vi "Areotech set positon.vi"(8 "error in (no error)":errorcluster, 10 "Parsed CMD":T1, 11 "AerotechStage in":refnum<class "AerotechStage.lvclass">) -> (0 "error out":errorcluster, 2 "new commands":string, 3 "AerotechStage out":refnum<class "AerotechStage.lvclass">)   [LabVIEW 2013, in "AerotechStage.lvclass"]
uses:
  AerotechStage.lvclass
  shared/parsed device cmd.ctl
  AerotechStage.lvclass/AerotechStage.ctl
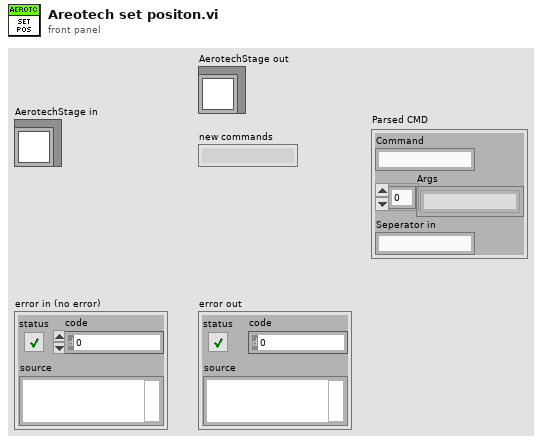
[diagram p1: front panel]
types:
  T1 = typedef "parsed device cmd.ctl" = cluster{"Command":string, "Args":string[], "Seperator in":string}
  T2 = typedef "OnOffTypeDef.ctl" = enum16{"off", "on"}
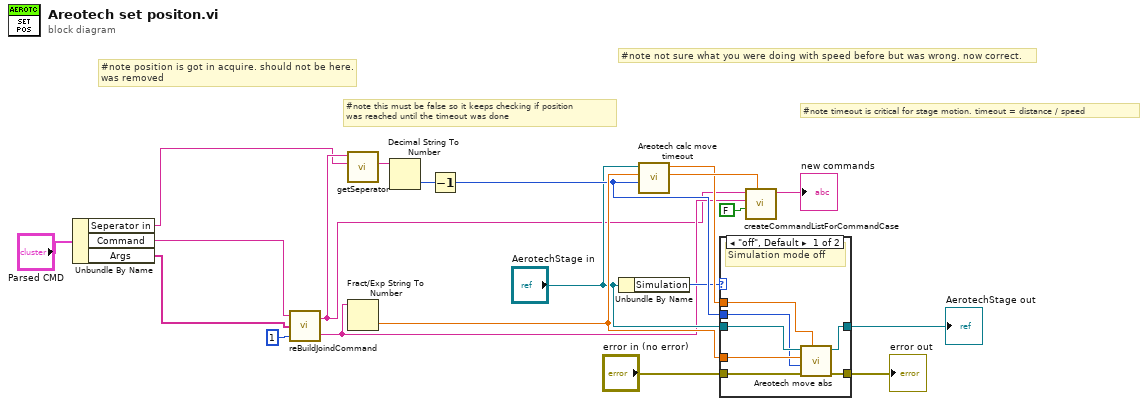
[diagram p0: block diagram]
diagram:
  # "#note position is got in acquire. should not be here.\nwas removed"
  # "#note not sure what you were doing with speed before but was wrong. now correct."
  # "#note timeout is critical for stage motion. timeout = distance / speed"
  # "#note this must be false so it keeps checking if position\nwas reached until the timeout was done"
  n1 = Unbundle By Name("Parsed CMD") -> ("Seperator in"=w2:string, "Command"=w3:string, "Args"=w1:string[])
  n2 = call "reBuildJoindCommand.vi"("number of group elements (0)"=1, "Args"=w1, "Command 2"=w3) -> ("Arg"=w9:string, "Command"=w7:string)
  n3 = call "getSeperator.vi"("Channel Seperator (\"\")"=w2, "Command"=w7) -> ("Channel"=w12:string)  [unwired: 8 in, 1 out]
  n4 = Fract/Exp String To Number(string=w9) -> (number=w18:dbl)  [unwired: 3 in, 1 out]
  n5 = Decimal String To Number(string=w12) -> (number=w11:i32)  [unwired: 2 in, 1 out]
  n6 = Decrement(x=w11) -> (x-1=w17:i32)
  n7 = Unbundle By Name("AerotechStage in") -> ("Simulation"=w10:T2)
  n8 = call "Areotech calc move timeout.vi"("Numeric in"=w17, "Position"=w18, "AerotechStage in"="AerotechStage in") -> ("Numeric out"=w20:dbl, "Value"=w19:dbl)  [unwired: 7 in]
  n9 = case shown="\"off\", Default" w10 {
    tunnel: w18 -> [w25 _]
    tunnel: "AerotechStage in" -> [w27 w28]
    tunnel: "error in (no error)" -> [w23 w29]
    tunnel: [w24 w29] -> w14
    tunnel: [w26 w28] -> w15
    tunnel: w17 -> [w22 _]
    tunnel: w19 -> [w21 _]
    frame "off", Default {
      # "Simulation mode off"
      n10 = call "Areotech move abs.vi"("speed"=w21, "error in (no error)"=w23, "stage index"=w22, "position"=w25, "AerotechStage in"=w27) -> ("error out"=w24:errorcluster, "AerotechStage out"=w26:refnum<class "AerotechStage.lvclass">)  [unwired: 5 in]
    }
    frame "on" {
      # "Simulation mode on"
    }
  }
  "AerotechStage out" <- w15
  "error out" <- w14
  n11 = call "createCommandListForCommandCase.vi"("timeout (optional)"=w20, "immediate Check (only once)"=FALSE, "setvalue"=w9, "command"=w7) -> ("new commands"=→"new commands":string)  [unwired: 7 in]
